vi "Convert Schedule to Sequence of SBlocks.vi"(3 "Schedule":refnum<class "Schedule.lvclass">) -> (0 "error out":errorcluster, 1 "Sequence of SBlocks":refnum<class "Sequence of SBlocks.lvclass">)   [LabVIEW 2020, in "CIRCUS_uServices.lvlib" / "Run Utilities.lvlib" / "Sequence of SBlocks.lvclass"]
uses:
  Sequence of SBlocks.lvclass
  Sequence of SBlocks.lvclass/Sequence of SBlocks.ctl
  Schedule/Schedule.lvclass
  Schedule Block/Schedule Block.lvclass
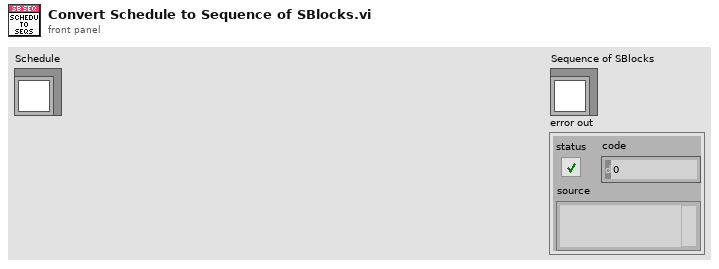
[diagram p1: front panel]
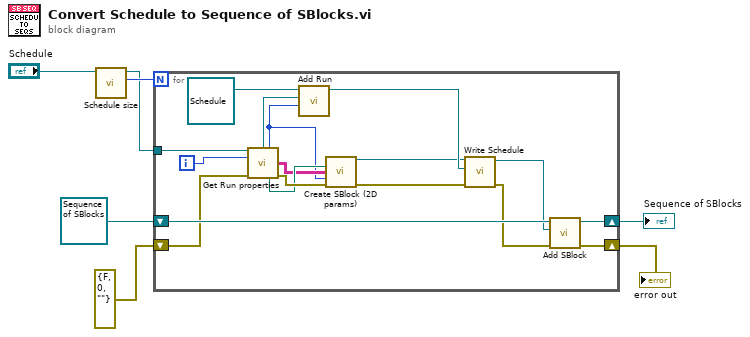
[diagram p0: block diagram]
diagram:
  n1 = call-dynamic "Schedule size.vi"("Schedule in"="Schedule") -> ("Size"=w6:i32, "Schedule out"=w3:refnum<class "Schedule.lvclass">)  [unwired: 8 in, 1 out]
  n2 = for {
    N: w6 -> [_]
    shift-right: [w19] -> w4
    shift-left: refnum<class "Sequence of SBlocks.lvclass"> refnum ("Run Utilities.lvlib:Sequence of SBlocks.lvclass") -> [w20]
    tunnel: w3 -> [w23]
    shift-right: [w18] -> w1
    shift-left: errorcluster {"status"=FALSE, "code"=0, "source"=""} ("error out") -> [w17]
    i -> [w22]
    n3 = call "Get Run properties.vi"("Schedule in"=w23, "index"=w22, "error in (no error)"=w17) -> ("Run Instance"=w15:refnum<class "Run Instance.lvclass">, "Repetitions"=w10:u32, "Parameters"=w11:string[][], "Script Path"=w21:path, "error out"=w24:errorcluster)  [unwired: 5 in, 3 out]
    n4 = call-dynamic "Add Run.vi"("Number of repetitions"=w10, "Run Instance"=w15, "Schedule in"=refnum<class "Schedule.lvclass"> refnum) -> ("Schedule out"=w13:refnum<class "Schedule.lvclass">)  [unwired: 7 in, 1 out]
    n5 = call "Create SBlock (2D params).vi"("Script Path"=w21, "Common Parameters"=w11, "Number of repetitions"=w10, "error in (no error)"=w24) -> ("Schedule Block out"=w9:refnum<class "Schedule Block.lvclass">, "error out"=w8:errorcluster)  [unwired: 9 in, 1 out]
    n6 = call-dynamic "Write Schedule.vi"("error in (no error)"=w8, "Schedule"=w13, "Schedule Block in"=w9) -> ("error out"=w16:errorcluster, "Schedule Block out"=w12:refnum<class "Schedule Block.lvclass">)  [unwired: 7 in]
    n7 = call-dynamic "Add SBlock.vi"("error in (no error)"=w16, "new SBlock"=w12, "Sequence of SBlocks in"=w20) -> ("error out"=w18:errorcluster, "Sequence of SBlocks out"=w19:refnum<class "Sequence of SBlocks.lvclass">)  [unwired: 7 in]
  }
  "Sequence of SBlocks" <- w4
  "error out" <- w1
